vi "Frisbee Drive Control.vi"(8 "Circle Info":cluster{dbl, dbl}, 9 "Vertical Constant":dbl=0.5, 10 "Horizontal Constant":dbl=0.9, 11 "Deadband":dbl=0.15) -> (2 "Right Drive":dbl, 3 "Left Drive":dbl)   [LabVIEW 2012]
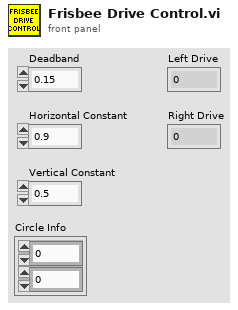
[diagram p1: front panel]
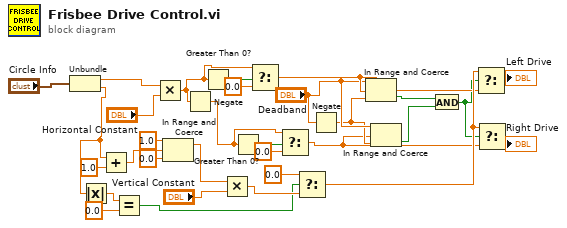
[diagram p0: block diagram]
diagram:
  n1 = Unbundle("Circle Info") -> (w2:dbl, w31:dbl)
  n2 = Absolute Value(x=w31) -> (abs(x)=w30:dbl)
  n3 = Add(x=w31, y=1.0) -> (x+y=w23:dbl)
  n4 = Equal?(x=w30, y=0.0) -> (x = y?=w26:bool)
  n5 = Multiply(x=w2, y="Horizontal Constant") -> (x*y=w5:dbl)
  n6 = In Range and Coerce(upper limit=1.0, x=w23, lower limit=0.0) -> (coerced(x)=w16:dbl)  [unwired: 1 out]
  n7 = Negate(x=w5) -> (-x=w9:dbl)
  n8 = Greater Than 0?(x=w5) -> (x > 0?=w4:bool)
  n9 = Multiply(x=w16, y="Vertical Constant") -> (x*y=w27:dbl)
  n10 = Greater Than 0?(x=w9) -> (x > 0?=w8:bool)
  n11 = Select(t=w5, s=w4, f=0.0) -> (s? t:f=w22:dbl)
  n12 = Select(t=w9, s=w8, f=0.0) -> (s? t:f=w19:dbl)
  n13 = Select(t=0.0, s=w26, f=w27) -> (s? t:f=w29:dbl)
  n14 = Negate(x="Deadband") -> (-x=w20:dbl)
  n15 = In Range and Coerce(upper limit="Deadband", x=w22, lower limit=w20) -> (In Range?=w17:bool)  [unwired: 1 out]
  n16 = In Range and Coerce(upper limit="Deadband", x=w19, lower limit=w20) -> (In Range?=w18:bool)  [unwired: 1 out]
  n17 = And(x=w17, y=w18) -> (x .and. y?=w10:bool)
  n18 = Select(t=w29, s=w10, f=w22) -> (s? t:f=→"Left Drive":dbl)
  n19 = Select(t=w29, s=w10, f=w19) -> (s? t:f=→"Right Drive":dbl)
